vi "GetCost.vi"(8 "error in (no error)":errorcluster, 11 "reference in":refnum<class "GetCostVisitor.lvclass">) -> (0 "error out":errorcluster, 2 "Cost String":string, 3 "reference in":refnum<class "GetCostVisitor.lvclass">)   [LabVIEW 2020, in "GetCostVisitor.lvclass"]
uses:
  GetCostVisitor.lvclass
  Equipment_class/Equipment.lvclass
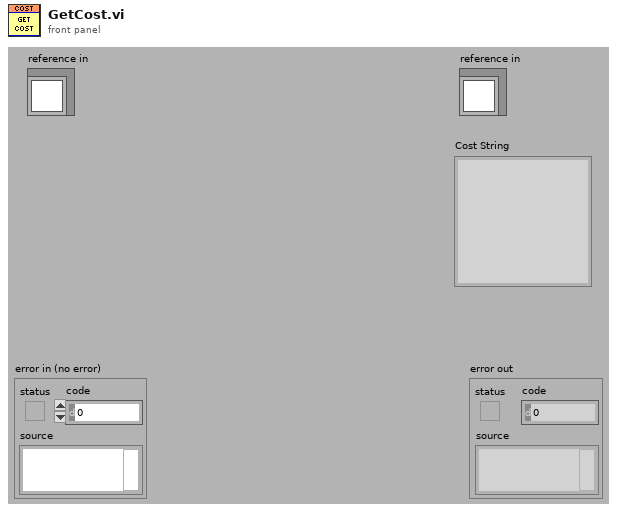
[diagram p1: front panel]
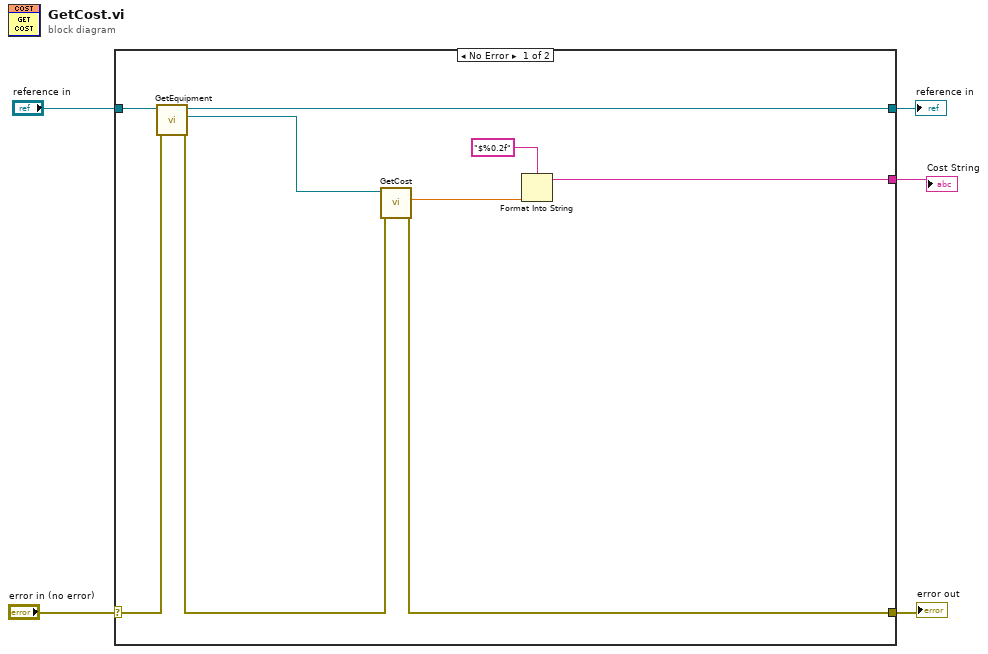
[diagram p0: block diagram]
diagram:
  n1 = case shown="No Error" "error in (no error)" {
    selector: "error in (no error)" -> [w13 w16]
    tunnel: [w9 w16] -> w4
    tunnel: [w12 w15] -> w2
    tunnel: "reference in" -> [w14 w15]
    tunnel: [w6 _] -> w1
    frame No Error {
      n2 = call-dynamic "GetEquipment.vi"("error in (no error)"=w13, "reference in"=w14) -> ("error out"=w10:errorcluster, "Equipment"=w11:refnum<class "Equipment.lvclass">, "reference out"=w12:refnum<class "GetCostVisitor.lvclass">)  [unwired: 7 in]
      n3 = call-dynamic "GetCost.vi"("error in (no error)"=w10, "reference in"=w11) -> ("error out"=w9:errorcluster, "Cost"=w8:dbl)  [unwired: 7 in, 1 out]
      n4 = Format Into String(format string="$%0.2f", w8) -> (resulting string=w6:string)  [unwired: 2 in, 1 out]
    }
    frame Error {
    }
  }
  "error out" <- w4
  "reference in" <- w2
  "Cost String" <- w1
